vi "HeaderAction.vi"(0 "InstrClass":refnum<class "SR530.lvclass"> caption="DNL_LabVIEW Object in", 11 "error in (no error)":errorcluster caption="entrée d'erreur (pas d'erreur)") -> (4 "InstrClassOut":refnum<class "SR530.lvclass"> caption="DNL_LabVIEW Object out", 6 "DataNames":string[](array[string]), 8 "Instr Name":string, 10 "HeaderString":string, 13 "ArrDisplayNames":string[](array[string]), 14 "DisplayNames":string[](array[string]), 15 "error out":errorcluster caption="sortie d'erreur")   [LabVIEW 2019, in "SR530.lvclass"]
uses:
  SR530.lvclass
  C:/Programmes LabView/LabScanV1A/DevicesClass/BaseDevice/BaseDevice.lvclass
  SR530.lvclass/SR530.ctl
  BaseDevice/BaseDevice.lvclass
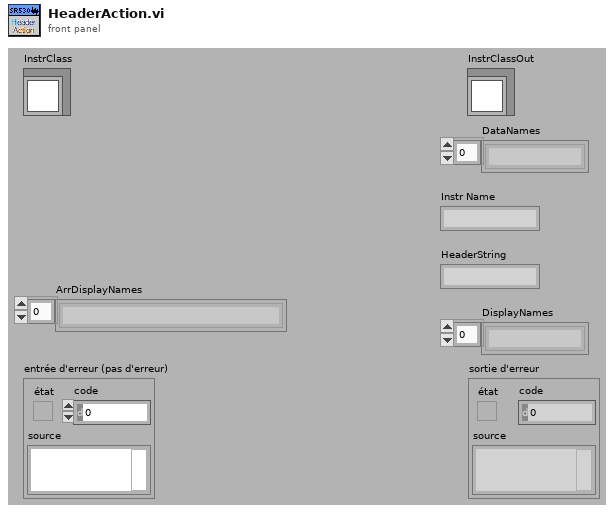
[diagram p1: front panel]
types:
  T1 = typedef "SR530.lvclass/SR530_Func.ctl" = enum16{"Read X & Y (V,V)", "Read Mag & Phase (V,°)", "Read X,Y,Mag & Phase (V,V,V,°)", "Read Analog Input (V)"}
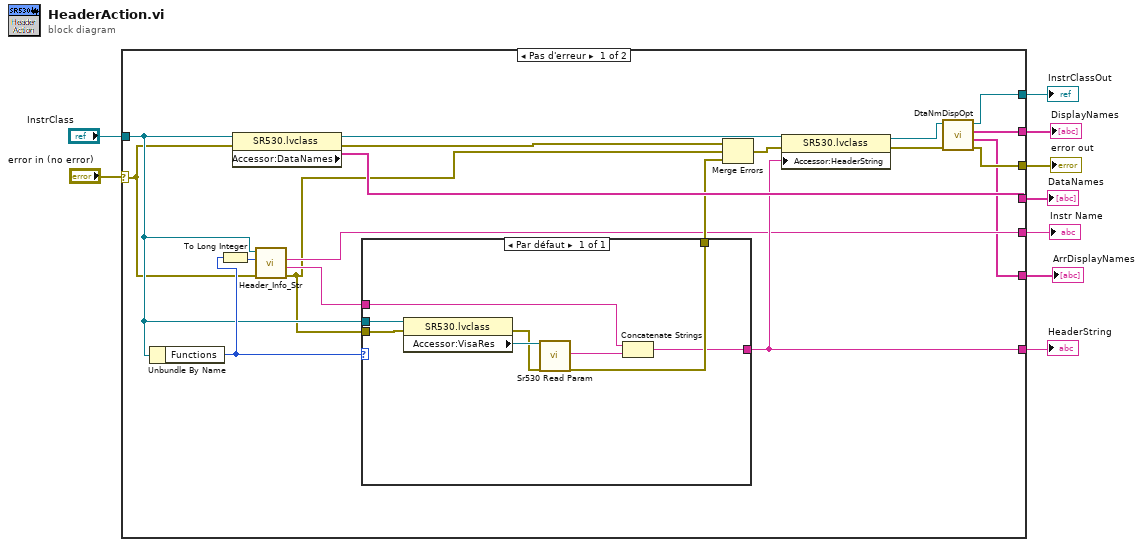
[diagram p0: block diagram]
diagram:
  n1 = case shown="Pas d'erreur" "error in (no error)" {
    selector: "error in (no error)" -> [w11 w37]
    tunnel: [w18 _] -> w8
    tunnel: [w28 _] -> w7
    tunnel: "InstrClass" -> [w15 w38]
    tunnel: [w24 w37] -> w5
    tunnel: [w23 w38] -> w3
    tunnel: [w14 _] -> w4
    tunnel: [w21 _] -> w2
    tunnel: [w10 _] -> w1
    frame No Error {
      n2 = Unbundle By Name(w15) -> ("Functions"=w16:T1)
      n3 = To Long Integer(number=w16) -> (32bit integer=w17:i32)
      n4 = property class="SR530.lvclass"(reference=w15, error in=w11) -> (reference out=w27:refnum<class "SR530.lvclass">, error out=w26:errorcluster, "Accessor:DataNames"=w28:string[])
      n5 = call-dynamic "Header_Info_Str.vi"("error in (no error)"=w11, "Functions"=w17, "DefaultDev in"=w15) -> ("error out"=w12:errorcluster, "HdrInfoStr"=w13:string, "InstrumentName"=w14:string)  [unwired: 5 in, 1 out]
      n6 = case shown="Par défaut" w16 {
        tunnel: w13 -> [w29]
        tunnel: w15 -> [w36]
        tunnel: w12 -> [w35]
        tunnel: [w32] -> w19
        tunnel: [w30] -> w18
        frame Par défaut {
          n7 = property class="SR530.lvclass"(reference=w36, error in=w35) -> (error out=w33:errorcluster, "Accessor:VisaRes"=w34:refnum<visa-resource-name>)  [unwired: 1 out]
          n8 = call <userlib>:"Sr530 Read Param.vi"("Ressource VISA"=w34, "error in (no error)"=w33) -> ("Params"=w31:string, "error out"=w32:errorcluster)  [unwired: 14 in, 2 out]
          n9 = Concatenate Strings(w29, w31) -> (w30:string)
        }
      }
      n10 = Merge Errors(w26, w12, w19) -> (w20:errorcluster)
      n11 = property class="SR530.lvclass"(reference=w27, error in=w20, "Accessor:HeaderString"=w18) -> (reference out=w22:refnum<class "SR530.lvclass">, error out=w25:errorcluster)
      n12 = call "DtaNmDispOpt.vi"("error in (no error)"=w25, "BaseDevice en entrée"=w22) -> ("error out"=w24:errorcluster, "ArrDisplayNames"=w10:string[], "DisplayNames"=w21:string[], "BaseDevice en sortie"=w23:refnum<class "SR530.lvclass">)  [unwired: 6 in]
    }
    frame Error {
    }
  }
  "error out" <- w5
  "InstrClassOut" <- w3
  "DataNames" <- w7
  "HeaderString" <- w8
  "Instr Name" <- w4
  "DisplayNames" <- w2
  "ArrDisplayNames" <- w1
